vi "GyroDrive.vi"() -> ()   [LabVIEW 2017]
uses:
  <vilib>/Rock Robotics/WPI/ThirdParty/Phoenix-LabVIEW/Motor Controller/Controls/CTRE_Phoenix_MotorControl_ControlMode.ctl
  <vilib>/Rock Robotics/WPI/Utilities/WPI_GetSetVariantRefNum.vi
  <vilib>/Rock Robotics/WPI/ThirdParty/Phoenix-LabVIEW/Pigeon IMU/CTRE_PigeonIMU_GetYPR.vi
panel:
  in  "Gyro Driver":bool
  in  "Pg":dbl
  in  "Ig":dbl
  in  "Contoller Constant":dbl
  in  "Gyro Point":bool
  in  "RC":bool
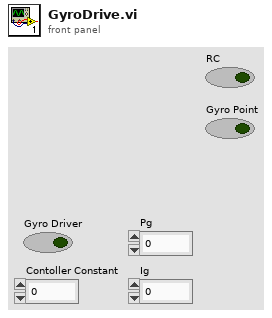
[diagram p1: front panel]
types:
  T1 = typedef "WPI_JoystickDevRef.ctl" = cluster{"Device":T2}
  T2 = typedef "WPI_JoystickDeviceEnum.ctl" = enum16{"USB 0", "USB 1", "USB 2", "USB 3", "USB 4", "USB 5"}
  T3 = typedef "WPI_MotorControlDeviceRef.ctl" = cluster{"DeviceStatus":errorcluster, "Type":T4, "PWM":cluster{"PWM Channel":T5, "DeadBand":T6}, "CAN":cluster{"Device Number":u8, "SetOutput VI Ref":variant, "GetOutput VI Ref":variant, "Enable VI Ref":variant, "Disable VI Ref":variant, "Data":variant}, "Invert":bool, "DIO PWM":cluster{"PWM \"Enable\" Channel":T5, "DIOChannel":T7, "PWM Rate":dbl}}
  T4 = typedef "WPI_MotorControlType.ctl" = enum16{"PWM", "CAN", "DIO PWM"}
  T5 = typedef "FPGA_DIOPWMChannel.ctl" = enum8{"PWM 0", "PWM 1", "PWM 2", "PWM 3", "PWM 4", "PWM 5", "PWM 6", "PWM 7", "PWM 8", "PWM 9", "PWM MXP 0", "PWM MXP 1", "PWM MXP 2", "PWM MXP 3", "PWM MXP 4", "PWM MXP 5", "PWM MXP 6", "PWM MXP 7", "PWM MXP 8", "PWM MXP 9", "Invalid"}
  T6 = typedef "WPI_PWMDeadband.ctl" = cluster{"Name":string, "maxPositivePwm":i32, "minPositivePwm":i32, "centerPwm":i32, "maxNegativePwm":i32, "minNegativePwm":i32, "angularRange":u16}
  T7 = typedef "FPGA_DIOChannel.ctl" = enum8{"DIO 0", "DIO 1", "DIO 2", "DIO 3", "DIO 4", "DIO 5", "DIO 6", "DIO 7", "DIO 8", "DIO 9", "DIO MXP 0", "DIO MXP 1", "DIO MXP 2", "DIO MXP 3", "DIO MXP 4", "DIO MXP 5", "DIO MXP 6", "DIO MXP 7", "DIO MXP 8", "DIO MXP 9", "DIO MXP 10", "DIO MXP 11", "DIO MXP 12", "DIO MXP 13", "DIO MXP 14", "DIO MXP 15", "SPI Port CS1", "SPI Port CS2", "SPI Port CS3", "SPI Port MISO", "SPI Port MOSI", "Invalid"}
  T8 = typedef "CTRE_PigeonIMU_DeviceRef.ctl" = cluster{"DeviceStatus":errorcluster, "Device Number":u8, "Type":T9, "Device ID":u32, "Handle":u64, "UsageFrame":u32, "Library Path":path}
  T9 = typedef "CTRE_PigeonIMU_ConnectionType.ctl" = u32
  T10 = typedef "CTRE_Phoenix_MotorControl_ControlMode.ctl" = u16
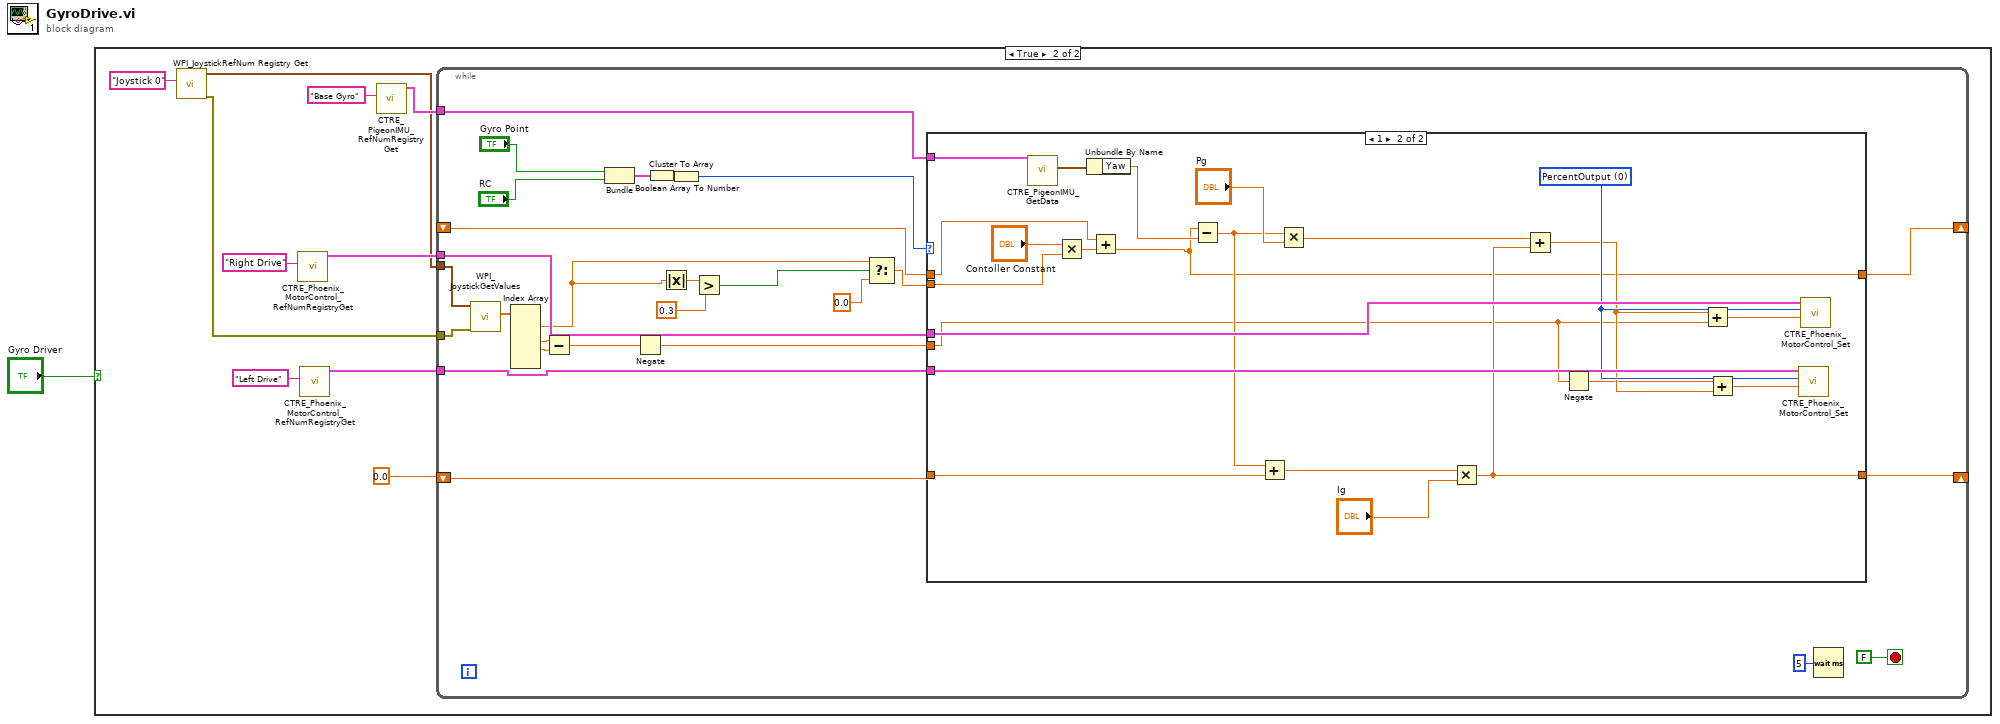
[diagram p0: block diagram]
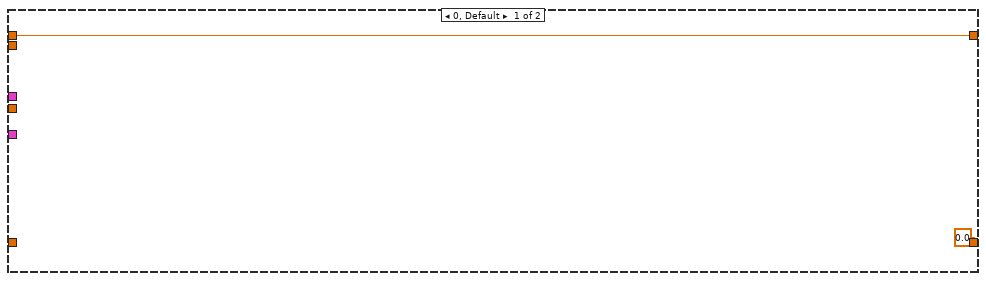
[diagram p3: hidden frame]
diagram:
  n1 = case shown="True" "Gyro Driver" {
    frame False {
    }
    frame True {
      n2 = call <vilib>:"WPI_JoystickRefNum Registry Get.vi"("refnum name"="Joystick 0") -> ("error out"=w3:errorcluster, "JoystickDevRef"=w2:T1)  [unwired: 1 in, 8 out]
      n3 = call "CTRE_Phoenix_MotorControl_RefNumRegistryGet.vi"("refnum name"="Right Drive") -> ("PhoenixMotorControlDevRef"=w6:T3)  [unwired: 9 in, 1 out]
      n4 = call "CTRE_Phoenix_MotorControl_RefNumRegistryGet.vi"("refnum name"="Left Drive") -> ("PhoenixMotorControlDevRef"=w5:T3)  [unwired: 9 in, 1 out]
      n5 = call "CTRE_PigeonIMU_RefNumRegistryGet.vi"("refnum name"="Base Gyro") -> ("PigeonIMUDevRef"=w10:T8)  [unwired: 9 in, 1 out]
      n6 = while {
        tunnel: w10 -> [w38]
        tunnel: w6 -> [w35]
        tunnel: w5 -> [w34]
        shift-right: [w32] -> _
        shift-left: 0.0 -> [w33]
        shift-right: [w26] -> _
        shift-left: _ -> [w25]
        tunnel: w3 -> [w23]
        tunnel: w2 -> [w22]
        stop <- FALSE stop-if-true
        n7 = call <vilib>:"WPI_JoystickGetValues.vi"("error in (no error)"=w23, "JoystickDevRef"=w22) -> ("Axes"=w24:dbl[])  [unwired: 5 in, 4 out]
        n8 = Index Array(array=w24) -> (element #1=w14:dbl, element #3=w21:dbl, element #4=w20:dbl)  [unwired: 6 in, 3 out]
        n9 = Subtract(x=w21, y=w20) -> (x-y=w19:dbl)
        n10 = Bundle("Gyro Point"="Gyro Point", "RC"="RC") -> (w31:cluster{"Gyro Point":bool, "RC":bool})  [unwired: 1 in]
        n11 = Negate(x=w19) -> (-x=w18:dbl)
        n12 = Cluster To Array(cluster=w31) -> (array=w29:bool[])
        n13 = Absolute Value(x=w14) -> (abs(x)=w15:dbl)
        n14 = Boolean Array To Number(Boolean array=w29) -> (number=w28:u32)
        n15 = Greater?(x=w15, y=0.3) -> (0:w12:bool)
        n16 = Select(t=w14, s=w12, f=0.0) -> (s? t:f=w17:dbl)
        n17 = case shown="1" w28 {
          tunnel: w38 -> [_ w56]
          tunnel: w35 -> [_ w61]
          tunnel: w34 -> [_ w60]
          tunnel: w33 -> [_ w54]
          tunnel: [0.0 w50] -> w32
          tunnel: [w39 w42] -> w26
          tunnel: w25 -> [w39 w41]
          tunnel: w17 -> [_ w43]
          tunnel: w18 -> [_ w45]
          frame 0, Default {
          }
          frame 1 {
            w59 = T10 0 items=["PercentOutput"=0, "Position"=1, "Velocity"=2, "Current"=3, "Follower"=5, "MotionProfile"=6, "MotionMagic"=7, "MotionMagicArc"=8, "MotionProfileArc"=10, "Disabled"=15] ("Control Mode")
            n18 = call-poly <vilib>:"CTRE_PigeonIMU_GetData.vi"("PigeonIMUDevRef"=w56) -> ("Yaw Pitch Roll"=w63:cluster{"Yaw":dbl, "Pitch":dbl, "Roll":dbl})  [unwired: 8 in, 2 out]
            n19 = Multiply(x="Contoller Constant", y=w43) -> (x*y=w49:dbl)
            n20 = Unbundle By Name(w63) -> ("Yaw"=w57:dbl)
            n21 = Add(x=w41, y=w49) -> (x+y=w42:dbl)
            n22 = Subtract(x=w42, y=w57) -> (x-y=w55:dbl)
            n23 = Add(x=w55, y=w54) -> (x+y=w53:dbl)
            n24 = Multiply(x=w55, y="Pg") -> (x*y=w58:dbl)
            n25 = Multiply(x=w53, y="Ig") -> (x*y=w50:dbl)
            n26 = Add(x=w58, y=w50) -> (x+y=w51:dbl)
            n27 = Negate(x=w45) -> (-x=w44:dbl)
            n28 = Add(x=w51, y=w45) -> (x+y=w47:dbl)
            n29 = Add(x=w44, y=w51) -> (x+y=w46:dbl)
            n30 = call "CTRE_Phoenix_MotorControl_Set.vi"("Output"=w46, "Control Mode"=w59, "PhoenixMotorControlDevRef"=w60) -> ()  [unwired: 7 in, 2 out]
            n31 = call "CTRE_Phoenix_MotorControl_Set.vi"("Output"=w47, "Control Mode"=w59, "PhoenixMotorControlDevRef"=w61) -> ()  [unwired: 7 in, 2 out]
          }
        }
        n32 = Wait (ms)(milliseconds to wait=u32 5) -> ()  [unwired: 1 out]
      }
    }
  }
